vi "Actor Core.vi"(8 "error in":errorcluster, 11 "Change Log in":refnum<class "Change Log.lvclass">) -> (0 "error out":errorcluster, 3 "Actor out":refnum<class "Actor.lvclass">)   [LabVIEW 2015, in "Change Log.lvlib" / "Change Log.lvclass"]
doc: "(<B>Filename</B>: Actor Framework.lvlib:Actor.lvclass:Actor Core.vi)\n\nReceives messages to the actor, reacts to them, and initiates any error handling that may shut the actor down.\n\nDescendant classes may override this VI to append parallel tasks for the actor to complete while it handles messages. Overrides use the Call Parent Method node."
uses:
  Change Log.lvclass
  UI Window/UI Window.lvclass
  <vilib>/ActorFramework/Actor/Actor.lvclass
  <vilib>/ActorFramework/Stop Msg/Stop Msg.lvclass
panel:
  in  "OK Button":bool
  out "Change Log Display":string
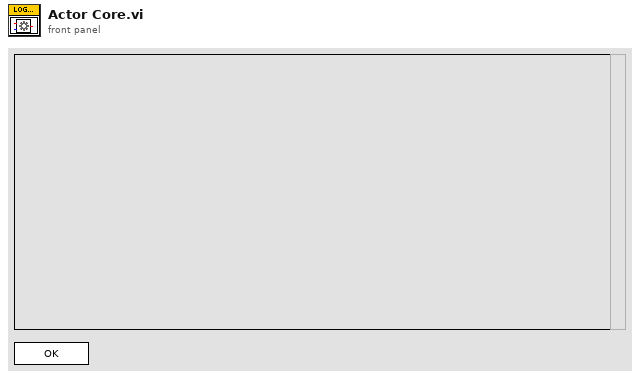
[diagram p1: front panel]
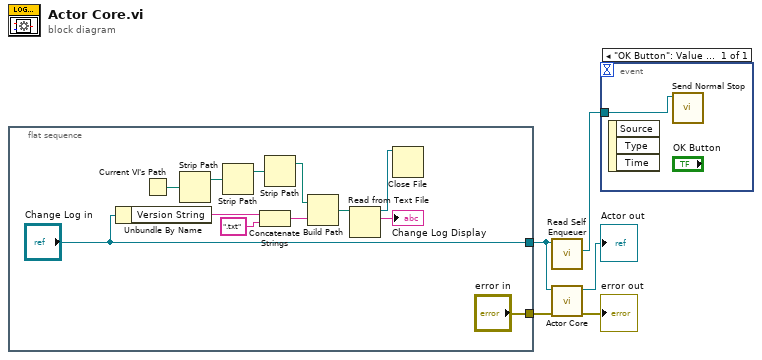
[diagram p0: block diagram]
diagram:
  n1 = flat-sequence {
    tunnel: ["error in"] -> w3
    tunnel: ["Change Log in"] -> w2
    frame #0 {
      n2 = Unbundle By Name("Change Log in") -> ("Version String"=w8:string)
      n3 = Current VI's Path() -> (path=w15:path)
      n4 = Strip Path(path=w15) -> (stripped path=w16:path)  [unwired: 1 out]
      n5 = Strip Path(path=w16) -> (stripped path=w11:path)  [unwired: 1 out]
      n6 = Concatenate Strings(w8, ".txt" ("name or relative path")) -> (w6:string)
      n7 = Strip Path(path=w11) -> (stripped path=w10:path)  [unwired: 1 out]
      n8 = Build Path(base path=w10, name or relative path=w6) -> (appended path=w12:path)
      n9 = Read from Text File(file (use dialog)=w12) -> (refnum out=w14:refnum<file>, text=→"Change Log Display":string)  [unwired: 3 in, 2 out]
      n10 = Close File(refnum=w14) -> ()  [unwired: 1 in, 2 out]
    }
  }
  n11 = call <vilib>:"Read Self Enqueuer.vi"("Actor"=w2) -> ("Self Enqueuer"=w1:refnum<class "Message Enqueuer.lvclass">)  [unwired: 10 in]
  n12 = call-parent "Actor Core.vi"("error in"=w3, "UI Window in"=w2) -> ("error out"=→"error out":errorcluster, "Actor out"=→"Actor out":refnum<class "Actor.lvclass">)  [unwired: 8 in]
  n13 = event shown="[0] \"OK Button\": Value Change" {
    selector: _ -> [_]
    dyn-events: _ -> [_]
    timeout: _ -> [_]
    tunnel: w1 -> [w18]
    event "OK Button": Value Change {
      n14 = event-data() -> ()  [unwired: 1 in, 3 out]
      n15 = call <vilib>:"Send Normal Stop.vi"("Message Enqueuer"=w18) -> ()  [unwired: 10 in, 1 out]
    }
  }
